vi "Read I8.vi"(11 "Event in":refnum<class "Event I8.lvclass">) -> (2 "I8":i8, 3 "Event out":refnum<class "Event I8.lvclass">)   [LabVIEW 2016, in "Event Source.lvlib" / "Event I8.lvclass"]
uses:
  Event I8.lvclass
  Event I8.lvclass/Event I8.ctl
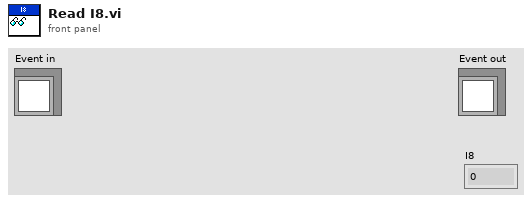
[diagram p1: front panel]
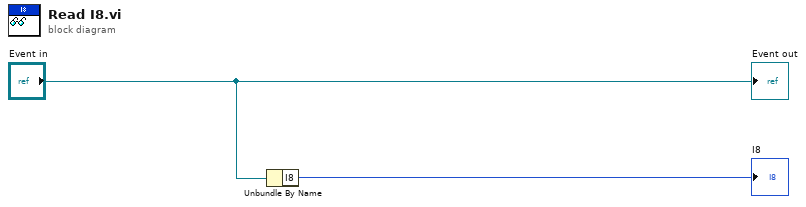
[diagram p0: block diagram]
diagram:
  n1 = Unbundle By Name("Event in") -> ("I8"=→"I8":i8)
  "Event out" <- "Event in"
